vi "HDF5_alarm_Cluster_to_Numeric.vi"(11 "TC 0":T1) -> (3 "f":dbl)   [LabVIEW 2018]
uses:
  Controls/Clusts/ErrorStatus.ctl
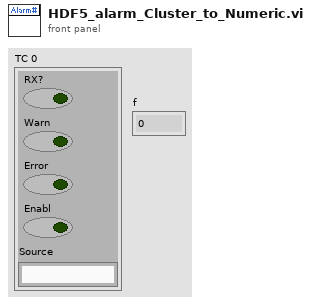
[diagram p1: front panel]
types:
  T1 = typedef "ErrorStatus.ctl" = cluster{"RX?":bool, "Warn":bool, "Error":bool, "Enabl":bool, "Source":string}
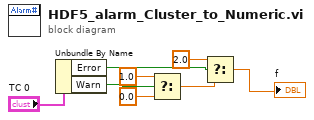
[diagram p0: block diagram]
diagram:
  n1 = Unbundle By Name("TC 0") -> ("Error"=w5:bool, "Warn"=w2:bool)
  n2 = Select(t=1.0, s=w2, f=0.0) -> (s? t:f=w6:dbl)
  n3 = Select(t=2.0, s=w5, f=w6) -> (s? t:f=→"f":dbl)
